vi "Configure Arbitrary Waveform Advanced.vi"(7 "Filter Mode (1: Step)":i32(ring)=1 items=["Normal", "Step", "Off"], 8 "error in (no error)":errorcluster, 9 "Advance Mode (0: Trigger)":i32(ring) items=["Trigger", "Sample Rate"], 10 "Channel (1: 1)":i32(ring)=1 items=["1"=1, "2"=2], 11 "VISA resource name":refnum<visa-resource-name>) -> (0 "error out":errorcluster, 3 "VISA resource name out":refnum<visa-resource-name>)   [LabVIEW 2018, in "Agilent 3352X Series.lvlib"]
doc: "Sets special parameters for arbitrary waveform, like advancing method, filtering settings and sample rate.\n\n<b>Note</b>:\nThis VI is intended to be used with Configure Arbitrary Waveform.VI to provide some advanced settings. Calling this VI only will not change current waveform function."
uses:
  <instrlib>/Agilent 3352X Series/Agilent 3352X Series.lvlib
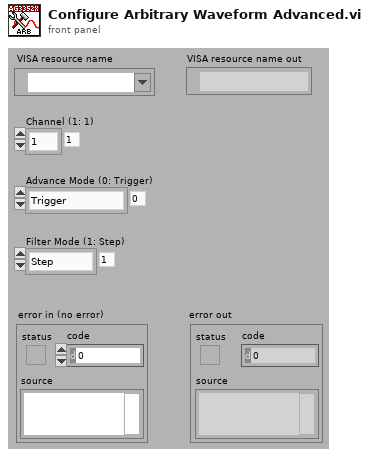
[diagram p1: front panel]
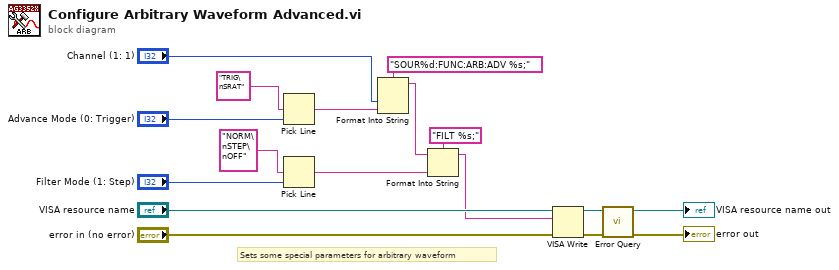
[diagram p0: block diagram]
diagram:
  # "Sets some special parameters for arbitrary waveform"
  n1 = Pick Line(multi-line string="TRIG\nSRAT", line index="Advance Mode (0: Trigger)") -> (output string=w13:string)  [unwired: 1 out]
  n2 = Pick Line(multi-line string="NORM\nSTEP\nOFF", line index="Filter Mode (1: Step)") -> (output string=w5:string)  [unwired: 1 out]
  n3 = Format Into String(format string="SOUR%d:FUNC:ARB:ADV %s;", "Channel (1: 1)", w13) -> (resulting string=w10:string)  [unwired: 2 in, 1 out]
  n4 = Format Into String(format string="FILT %s;", initial string=w10, w5) -> (resulting string=w6:string)  [unwired: 1 in, 1 out]
  n5 = VISA Write(VISA resource name="VISA resource name", write buffer=w6, error in (no error)="error in (no error)") -> (VISA resource name out=w4:refnum<visa-resource-name>, error out=w3:errorcluster)  [unwired: 1 out]
  n6 = call <instrlib>:"Error Query.vi"("error in (no error)"=w3, "VISA resource name"=w4) -> ("error out"=→"error out":errorcluster, "VISA resource name out"=→"VISA resource name out":refnum<visa-resource-name>)  [unwired: 8 out]
